vi "6.vi"(8 "error in (no error)":errorcluster, 9 "File Property Name":string, 10 "File Property Name":string, 11 "String in":string) -> (0 "error out":errorcluster, 3 "String out":string)   [LabVIEW 2015]
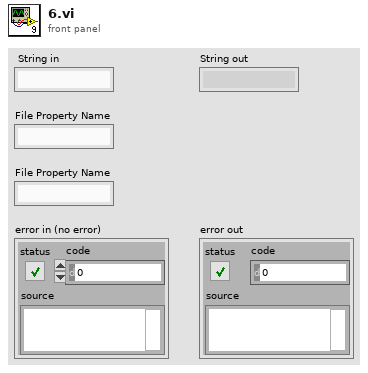
[diagram p1: front panel]
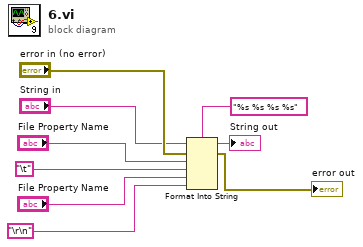
[diagram p0: block diagram]
diagram:
  n1 = Format Into String(format string="%s %s %s %s", initial string="String in", error in="error in (no error)", "File Property Name", "\t", "File Property Name", "\r\n") -> (resulting string=→"String out":string, error out=→"error out":errorcluster)
